vi "Purge Queue.vi"(8 "error in (no error)":errorcluster, 11 "SQS in":refnum<class "Queue.lvclass">) -> (0 "error out":errorcluster, 3 "SQS out":refnum<class "Queue.lvclass">)   [LabVIEW 2015, in "NI_AWS_SQS.lvlib" / "Queue.lvclass"]
doc: "Deletes the messages in a queue specified by the QueueURL parameter.\n\nImportant\nWhen you use the PurgeQueue action, you can't retrieve a message deleted from a queue.\nWhen you purge a queue, the message deletion process takes up to 60 seconds. All messages sent to the queue before calling the PurgeQueue action are deleted. Messages sent to the queue while it is being purged might be deleted. While the queue is being purged, messages sent to the queue before PurgeQueue is called might be received, but are deleted within the next minute."
uses:
  Queue.lvclass
  Core/HTTP Request/Name Value Pair.ctl
  Core/HTTP Request/Request Options.ctl
  Core/HTTP Request/Region handling.ctl
  Core/HTTP Request/URL formatting.ctl
  Queue.lvclass/Queue.ctl
  Read Account Number.vi
  Read Name.vi
  Core/HTTP Request/HTTP Request.lvclass
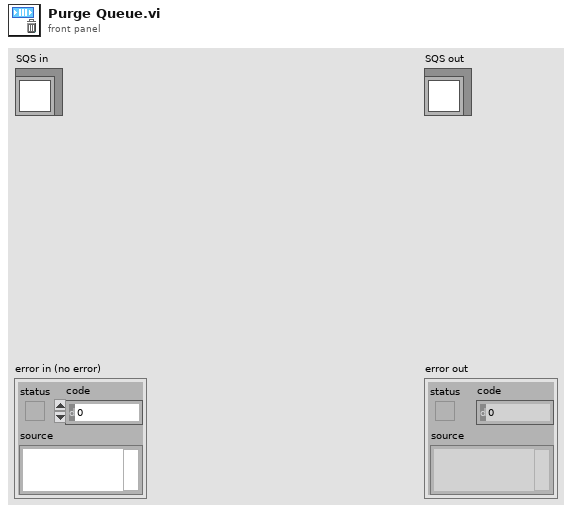
[diagram p1: front panel]
types:
  T1 = typedef "NI_AWS_Core.lvlib/HTTP Request.lvclass/Request Options.ctl" = cluster{"request headers":T2[], "request parameters":T2[], "request body":string, "region handling":T3, "URL formatting":T4}
  T2 = typedef "NI_AWS_Core.lvlib/HTTP Request.lvclass/Name Value Pair.ctl" = cluster{"name":string, "value":string}
  T3 = typedef "NI_AWS_Core.lvlib/HTTP Request.lvclass/Region handling.ctl" = enum16{"use region everywhere", "use region (authentication only)", "use region (URL only)", "ignore region everwhere"}
  T4 = typedef "NI_AWS_Core.lvlib/HTTP Request.lvclass/URL formatting.ctl" = enum16{"region-", "region."}
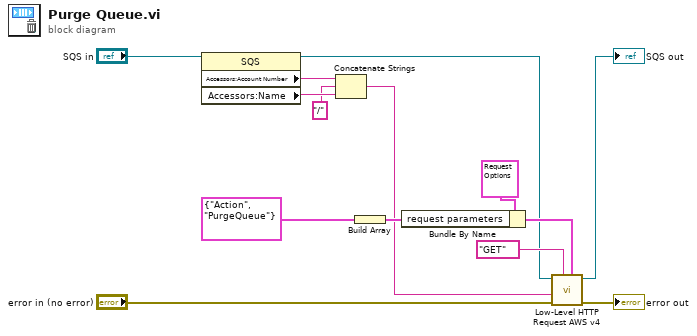
[diagram p0: block diagram]
diagram:
  n1 = property class="SQS"(reference="SQS in") -> (reference out=w2:refnum<class "Queue.lvclass">, "Accessors:Account Number"=w9:string, "Accessors:Name"=w8:string)  [unwired: 1 in, 1 out]
  n2 = Concatenate Strings(w9, "/", w8) -> (w6:string)
  n3 = Build Array(T2 {"name"="Action", "value"="PurgeQueue"} ("Cluster")) -> (w10:T2[])
  n4 = Bundle By Name(cluster=T1 {"request headers"=[], "request parameters"=[{"name"="Action", "value"="ListQueues"}], "request body"="", "region handling"=enum."use region everywhere", "URL formatting"=enum."region."} ("Request Options"), "request parameters"=w10) -> (w3:T1)
  n5 = call "Low-Level HTTP Request AWS v4.vi"("Request Options"=w3, "HTTP-Verb"="GET", "error in (no error)"="error in (no error)", "URL Suffix"=w6, "AWS Core in"=w2) -> ("error out"=→"error out":errorcluster, "AWS Core out"=→"SQS out":refnum<class "Queue.lvclass">)  [unwired: 3 in, 2 out]
